vi "GetRxPendingMsg.vi"(8 "error in (no error)":errorcluster, 11 "National Instruments USB-8473 Adapter Class in":refnum<class "National Instruments USB-8473 Adapter Class.lvclass">) -> (0 "error out":errorcluster, 2 "Value":i32, 3 "National Instruments USB-8473 Adapter Class out":refnum<class "National Instruments USB-8473 Adapter Class.lvclass">)   [LabVIEW 2011, in "National Instruments USB-8473 Adapter Class.lvclass"]
uses:
  National Instruments USB-8473 Adapter Class.lvclass
  Generic CAN Adapter/GenericCanAdapterClass.lvclass
  National Instruments USB-8473 Adapter Class.lvclass/National Instruments USB-8473 Adapter Class.ctl
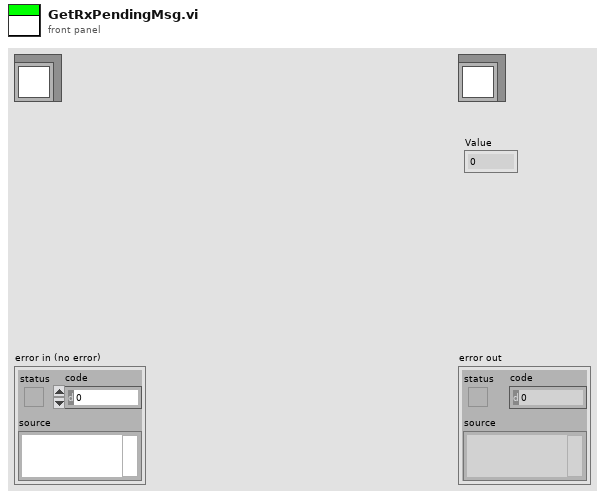
[diagram p1: front panel]
types:
  T1 = typedef "xobjhandle.ctl" = u32
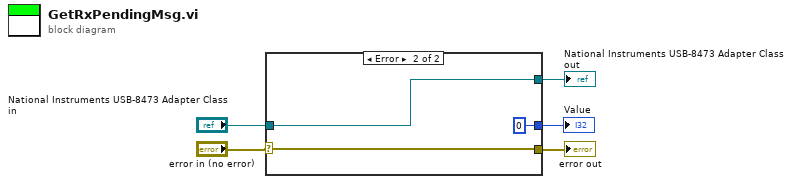
[diagram p0: block diagram]
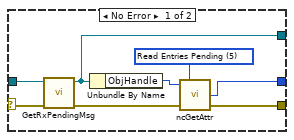
[diagram p2: hidden frame]
diagram:
  n1 = case shown="Error" "error in (no error)" {
    selector: "error in (no error)" -> [w6 w16]
    tunnel: "National Instruments USB-8473 Adapter Class in" -> [w13 w14]
    tunnel: [w10 w14] -> w4
    tunnel: [w8 w16] -> w3
    tunnel: [w7 u32 0 ("AttrValue")] -> w2
    frame No Error {
      w12 = u32 5 items=["(reserved)", "Protocol Version", "Software Version", "Object State", "(reserved)", "Read Entries Pending", "Write Entries Pending", "ReadMult Size for Notification", "Listen Only?", "Self Reception?", "Transmit Error Counter", "Receive Error Counter", "Single Shot Transmit?", "Series 2 Filter Mode", "Series 2 Mask", "Series 2 Comparator", "Serial Number", "Form Factor", "Series", "Transceiver Type", "Interface Number", "Series 2 Error/Arb Capture", "Transceiver Mode", "Transceiver External Outputs", "Transceiver External Inputs", "Start Trigger Behavior", "Log Comm Warnings", "User RTSI Frame", "Transmit Mode", "Log Start Trigger?", "Timestamp Format", "Master Timebase Rate", "Virtual Bus Timing"] ("AttrId")
      n2 = call-parent "GetRxPendingMsg.vi"("error in (no error)"=w6, "GenericCanAdapterClass in"=w13) -> ("error out"=w11:errorcluster, "GenericCanAdapterClass out"=w10:refnum<class "National Instruments USB-8473 Adapter Class.lvclass">)  [unwired: 7 in, 1 out]
      n3 = Unbundle By Name(w10) -> ("ObjHandle"=w9:T1)
      n4 = call <vilib>:"ncGetAttr.vi"("Error in"=w11, "AttrId"=w12, "ObjHandle in"=w9) -> ("Error out"=w8:errorcluster, "AttrValue"=w7:u32)  [unwired: 1 out]
    }
    frame Error {
    }
  }
  "error out" <- w3
  "National Instruments USB-8473 Adapter Class out" <- w4
  "Value" <- w2
